vi "Download program temp.vi"(8 "error in (no error)":errorcluster, 9 "Segment":dbl=6.0, 10 "Address":dbl=1.0, 11 "VISA resource name (IN)":refnum<visa-resource-name>) -> (0 "error out":errorcluster, 2 "Downloaded Temp.  data":dbl, 3 "VISA resource name (OUT)":refnum<visa-resource-name>)   [LabVIEW 2010, in "Yudian AI508.lvlib"]
uses:
  <instrlib>/Yudian AI508/Yudian AI508.lvlib
panel:
  out "Recieved Raw Data":string
  out "Data buffer":string
  out "Digital shift":i32
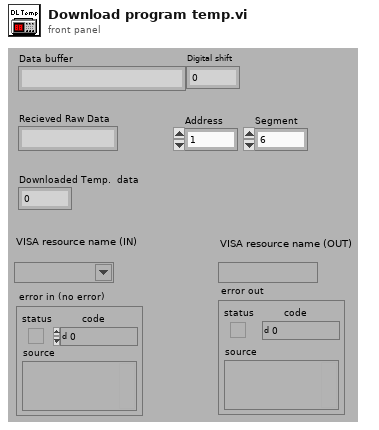
[diagram p1: front panel]
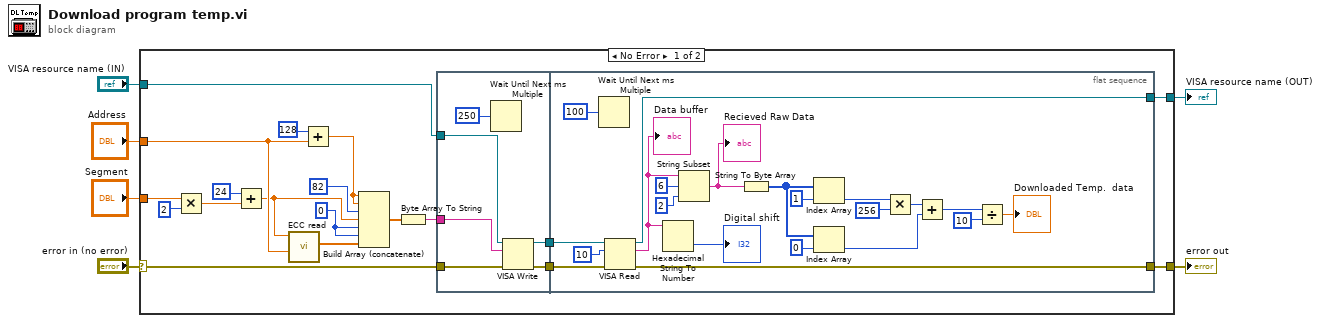
[diagram p0: block diagram]
diagram:
  n1 = case shown="No Error" "error in (no error)" {
    selector: "error in (no error)" -> [w20 w54]
    tunnel: [w22 w54] -> w6
    tunnel: [w23 w53] -> w5
    tunnel: "VISA resource name (IN)" -> [w21 w53]
    tunnel: "Segment" -> [w11 _]
    tunnel: "Address" -> [w14 _]
    frame No Error {
      w12 = 0
      n2 = Multiply(x=w11, y=2) -> (x*y=w8:dbl)
      n3 = Add(x=24, y=w8) -> (x+y=w7:dbl)
      n4 = call <instrlib>:"ECC read.vi"("Address"=w14, "Parameter code"=w7) -> ("Data array"=w13:dbl[])  [unwired: 9 in]
      n5 = Add(x=128, y=w14) -> (x+y=w19:dbl)
      n6 = Build Array (concatenate)(w19, w19, 82, w7, w12, w12, w13) -> (w16:dbl[])
      n7 = Byte Array To String(unsigned byte array=w16) -> (string=w15:string)
      n8 = flat-sequence {
        tunnel: w20 -> [w31]
        tunnel: w21 -> [w28]
        tunnel: [w30] -> w25
        tunnel: [w29] -> w24
        tunnel: w15 -> [w26]
        tunnel: w25 -> [w38]
        tunnel: w24 -> [w37]
        tunnel: [w35] -> w23
        tunnel: [w34] -> w22
        frame #0 {
          n9 = Wait Until Next ms Multiple(millisecond multiple=250) -> ()  [unwired: 1 out]
          n10 = VISA Write(VISA resource name=w28, write buffer=w26, error in (no error)=w31) -> (VISA resource name out=w29:refnum<visa-resource-name>, error out=w30:errorcluster)  [unwired: 1 out]
        }
        frame #1 {
          n11 = Wait Until Next ms Multiple(millisecond multiple=100) -> ()  [unwired: 1 out]
          n12 = VISA Read(VISA resource name=w37, byte count=u32 10 ("字节总数"), error in (no error)=w38) -> (VISA resource name out=w35:refnum<visa-resource-name>, read buffer=w40:string, error out=w34:errorcluster)  [unwired: 1 out]
          "Data buffer" <- w40
          n13 = Hexadecimal String To Number(string=w40) -> (number=→"Digital shift":u32)  [unwired: 3 out]
          n14 = String Subset(string=w40, offset (0)=6 ("length (rest)"), length (rest)=2 ("length (rest)")) -> (substring=w50:string)
          "Recieved Raw Data" <- w50
          n15 = String To Byte Array(string=w50) -> (unsigned byte array=w48:u8[])
          n16 = Index Array(array=w48, index=1) -> (element=w47:u8)
          n17 = Index Array(array=w48, index=0) -> (element=w44:u8)
          n18 = Multiply(x=w47, y=u16 256) -> (x*y=w45:u16)
          n19 = Add(x=w45, y=w44) -> (x+y=w43:u16)
          n20 = Divide(x=w43, y=u16 10) -> (x/y=→"Downloaded Temp.  data":dbl)
        }
      }
    }
    frame Error {
    }
  }
  "error out" <- w6
  "VISA resource name (OUT)" <- w5
